vi "Start Command.vi"(8 "error in (no error)":errorcluster, 11 "Command in":refnum<class "EL-Go To Height.lvclass">) -> (0 "error out":errorcluster, 3 "Command out":refnum<class "EL-Go To Height.lvclass">)   [LabVIEW 2014, in "Elevator.lvlib" / "EL-Go To Height.lvlib" / "EL-Go To Height.lvclass"]
uses:
  EL-Go To Height.lvclass
  EL-Go To Height Messages/Current Elevator State Msg/Current Elevator State Msg.lvclass
  Elevator Messages/Request Current State Msg/Request Current State Msg.lvclass
  <vilib>/ActorFramework/Actor/Actor.lvclass/Actor.ctl
  <vilib>/ActorFramework/Message Enqueuer/Message Enqueuer.lvclass/Message Enqueuer.ctl
  EL-Go To Height.lvclass/EL-Go To Height.ctl
  Elevator Messages/Request Current State Msg/Request Current State Msg.lvclass/Request Current State Msg.ctl
  <vilib>/ActorFramework/Message Enqueuer/Init from Existing Queue.vi
  <vilib>/ActorFramework/Message Enqueuer/Enqueue.vi
  <vilib>/ActorFramework/Message Priority Queue/Priority Enqueue.vi
  Robot Actor Framework/Command Actor/Command Actor Class/Command Actor.lvclass
  <vilib>/ActorFramework/Message Enqueuer/Message Enqueuer.lvclass
  EL-Go To Height Messages/Go To Assessing Msg/Go To Assessing Msg.lvclass
  <vilib>/ActorFramework/Actor/Actor.lvclass
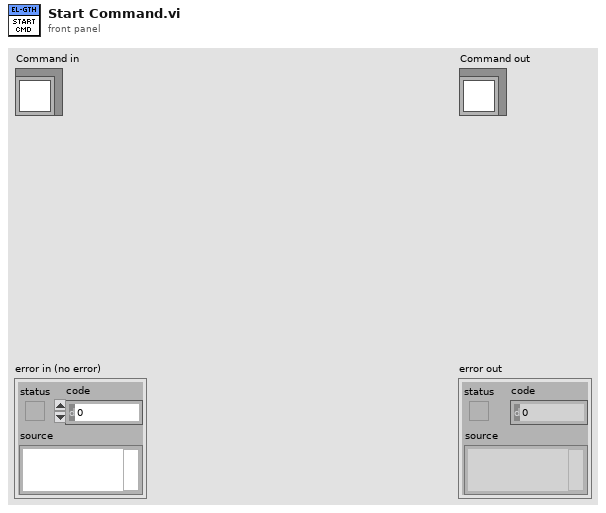
[diagram p1: front panel]
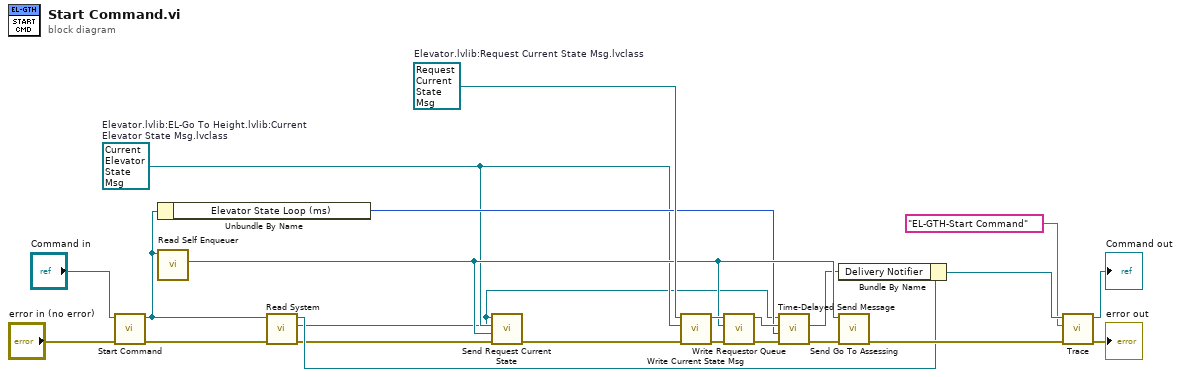
[diagram p0: block diagram]
diagram:
  w21 = refnum<class "Request Current State Msg.lvclass"> refnum  # Elevator.lvlib:Request Current State Msg.lvclass
  w6 = refnum<class "Current Elevator State Msg.lvclass"> refnum  # Elevator.lvlib:EL-Go To Height.lvlib:Current Elevator State Msg.lvclass
  n1 = call-parent "Start Command.vi"("error in (no error)"="error in (no error)", "Command in"="Command in") -> ("error out"=w2:errorcluster, "Command out"=w5:refnum<class "EL-Go To Height.lvclass">)  [unwired: 8 in]
  n2 = Unbundle By Name(w5) -> ("Elevator State Loop (ms)"=w16:u32)
  n3 = call <vilib>:"Read Self Enqueuer.vi"("Actor"=w5) -> ("Self Enqueuer"=w18:refnum<class "Message Enqueuer.lvclass">)  [unwired: 10 in]
  n4 = call-dynamic "Read System.vi"("error in (no error)"=w2, "Command in"=w5) -> ("error out"=w1:errorcluster, "Actor Framework:Message Enqueuer"=w3:refnum<class "Message Enqueuer.lvclass">, "Command out"=w4:refnum<class "EL-Go To Height.lvclass">)  [unwired: 7 in]
  n5 = call "Send Request Current State.vi"("error in (no error)"=w1, "Requestor Queue"=w18, "Elevator.lvlib:Current State Msg.lvclass"=w6, "Message Enqueuer"=w3) -> ("error out"=w9:errorcluster)  [unwired: 6 in, 1 out]
  n6 = call-dynamic "Write Current State Msg.vi"("error in (no error)"=w9, "Elevator.lvlib:Current State Msg.lvclass"=w6, "Request Current State Msg in"=w21) -> ("error out"=w8:errorcluster, "Request Current State Msg out"=w20:refnum<class "Request Current State Msg.lvclass">)  [unwired: 7 in]
  n7 = call-dynamic "Write Requestor Queue.vi"("error in (no error)"=w8, "Actor Framework:Message Enqueuer"=w18, "Request Current State Msg in"=w20) -> ("error out"=w7:errorcluster, "Request Current State Msg out"=w19:refnum<class "Request Current State Msg.lvclass">)  [unwired: 7 in]
  n8 = call <vilib>:"Time-Delayed Send Message.vi"("error in (no error)"=w7, "Milliseconds To Wait"=w16, "Message"=w19, "Message Enqueuer"=w3) -> ("error out"=w17:errorcluster, "Delivery Notifier"=w15:refnum<notifier>)  [unwired: 6 in]
  n9 = Bundle By Name(cluster=w4, "Delivery Notifier"=w15) -> (w12:refnum<class "EL-Go To Height.lvclass">)
  n10 = call "Send Go To Assessing.vi"("error in (no error)"=w17, "Message Enqueuer"=w18) -> ("error out"=w14:errorcluster)  [unwired: 8 in, 1 out]
  n11 = call-dynamic "Trace.vi"("error in (no error)"=w14, "Command Action"="EL-GTH-Start Command", "Command Actor in"=w12) -> ("error out"=→"error out":errorcluster, "Command Actor out"=→"Command out":refnum<class "EL-Go To Height.lvclass">)  [unwired: 7 in]
